vi "LoadFromINI.vi"(8 "error in (no error)":errorcluster, 10 "Path Control":path, 11 "reference in":refnum<class "NISync.lvclass">) -> (0 "error out":errorcluster, 3 "reference out":refnum<class "NISync.lvclass">)   [LabVIEW 2019, in "NISync.lvclass"]
uses:
  NISync.lvclass
  <vilib>/Utility/config.llb/NI_LVConfig.lvlib
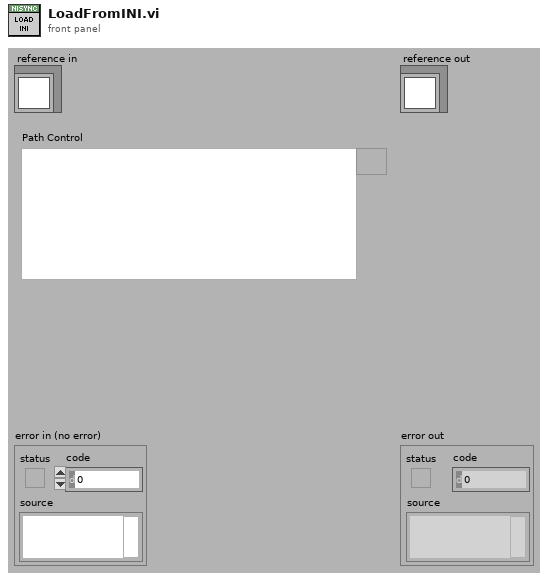
[diagram p1: front panel]
types:
  T1 = typedef "NISync.lvclass/ObjectAttributesRef.ctl" = refnum<data-value>
  T2 = typedef "NISync.lvclass/ObjectAttributes.ctl" = cluster{"Timing module":tag, "mode":enum16{"None", "Export trig", "Import trig"}, "Module terminal":string, "PXI line":string}
  T3 = typedef "NI_LVConfig.lvlib/Config Data RefNum.ctl" = refnum<k1>
  T4 = cluster{"mode":enum16{"None", "Export trig", "Import trig"}, "Module terminal":string, "PXI line":string}
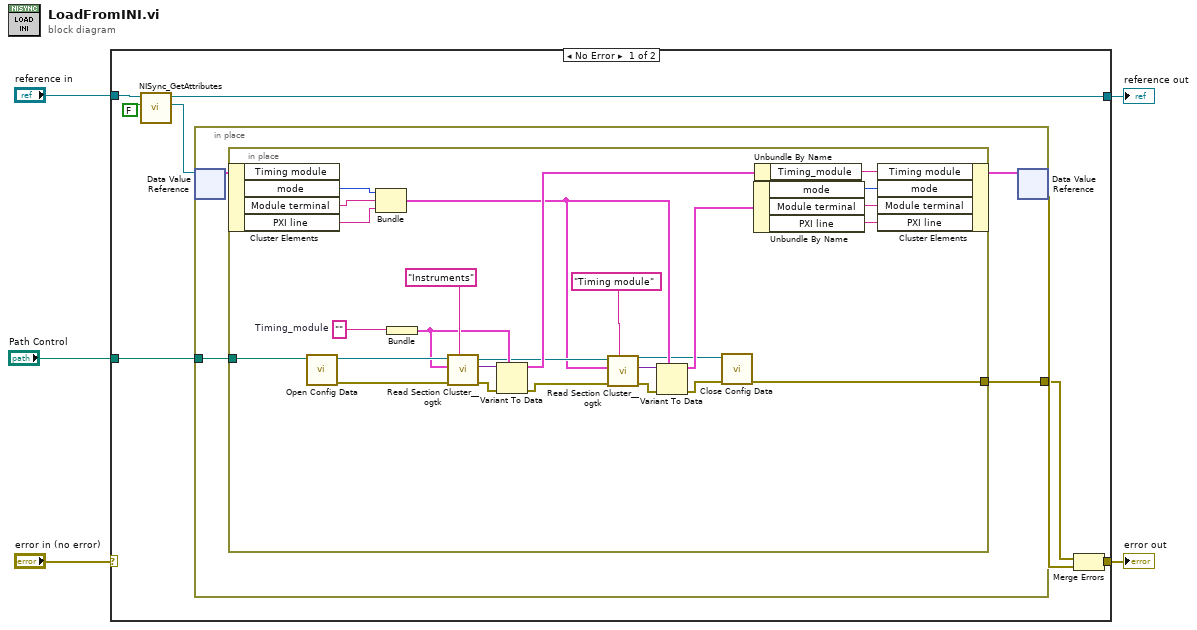
[diagram p0: block diagram]
diagram:
  n1 = case shown="No Error" "error in (no error)" {
    selector: "error in (no error)" -> [_ w45]
    tunnel: [w13 w45] -> w4
    tunnel: [w9 w44] -> w2
    tunnel: "reference in" -> [w11 w44]
    tunnel: "Path Control" -> [w7 _]
    frame No Error {
      n2 = call "NISync_GetAttributes.vi"("return data? (T)"=FALSE, "reference in"=w11) -> ("attributes ref"=w8:T1, "reference out"=w9:refnum<class "NISync.lvclass">)  [unwired: 6 in, 2 out]
      n3 = in-place {
        in-place-border: w7 -> [w15]
        in-place-border: [w14] -> w6
        n4 = in-place-dvr #1(w8) -> (w16:T2)  [unwired: 1 out]
        n5 = in-place {
          in-place-border: w15 -> [w43]
          in-place-border: [w18] -> w14
          w39 = ""  # Timing_module
          n6 = in-place-cluster #2(w16) -> ("mode"=w28:enum16{"None", "Export trig", "Import trig"}, "Module terminal"=w27:string, "PXI line"=w26:string)  [unwired: 1 out]
          n7 = call <vilib>:"Open Config Data.vi"("configuration file path"=w43) -> ("error out"=w41:errorcluster, "refnum"=w42:T3)  [unwired: 8 in, 1 out]
          n8 = Bundle("mode"=w28, "Module terminal"=w27, "PXI line"=w26) -> (w25:T4)  [unwired: 1 in]
          n9 = Bundle("Timing_module"=w39) -> (w36:cluster{"Timing_module":string})  [unwired: 1 in]
          n10 = call <userlib>:"Read Section Cluster__ogtk.vi"("section (optional)"="Instruments", "error in (no error)"=w41, "Section Formatted Cluster Type"=w36, "refnum"=w42) -> ("error out"=w38:errorcluster, "Section Formatted Cluster"=w37:variant, "dup refnum"=w30:T3)  [unwired: 3 in, 2 out]
          n11 = Variant To Data(error in=w38, type=w36, Variant=w37) -> (data=w35:cluster{"Timing_module":string}, error out=w31:errorcluster)
          n12 = call <userlib>:"Read Section Cluster__ogtk.vi"("section (optional)"="Timing module", "error in (no error)"=w31, "Section Formatted Cluster Type"=w25, "refnum"=w30) -> ("error out"=w32:errorcluster, "Section Formatted Cluster"=w33:variant, "dup refnum"=w20:T3)  [unwired: 3 in, 2 out]
          n13 = Variant To Data(error in=w32, type=w25, Variant=w33) -> (data=w24:T4, error out=w19:errorcluster)
          n14 = call <vilib>:"Close Config Data.vi"("error in (no error)"=w19, "refnum"=w20) -> ("error out"=w18:errorcluster)  [unwired: 8 in, 1 out]
          n15 = Unbundle By Name(w24) -> ("mode"=w23:enum16{"None", "Export trig", "Import trig"}, "Module terminal"=w22:string, "PXI line"=w21:string)
          n16 = Unbundle By Name(w35) -> ("Timing_module"=w34:string)
          n17 = in-place-cluster #2("Timing module"=w34, "mode"=w23, "Module terminal"=w22, "PXI line"=w21) -> (w17:T2)
        }
        n18 = in-place-dvr #1(w17) -> (w12:errorcluster)  [unwired: 1 out]
      }
      n19 = Merge Errors(w6, w12) -> (w13:errorcluster)
    }
    frame Error {
    }
  }
  "error out" <- w4
  "reference out" <- w2
